vi "TestResult_Init.vi"(8 "error in (no error)":errorcluster, 9 "testStartedEventRef":refnum<user-event>, 10 "resultStatusChangedEventRef":refnum<user-event>, 11 "TestResult in":refnum<class "TestResult.lvclass">) -> (0 "error out":errorcluster, 3 "TestResult out":refnum<class "TestResult.lvclass">)   [LabVIEW 2013, in "TestResult.lvclass"]
uses:
  TestResult.lvclass
  resultStatusChanged--Cluster.ctl
  resultStatus--enum.ctl
  testStarted--Cluster.ctl
  private/testsRun.ctl
  private/shouldStop.ctl
  private/errors.ctl
  private/error.ctl
  private/failure.ctl
  TestResult.lvclass/TestResult.ctl
panel:
  # "JKI VI Tester for LabVIEW\nhttp://jkisoft.com/vi-tester\nCopyright (C) 2007-2009, JKI <info@jkisoft.com>\nALL RIGHTS RESERVED"
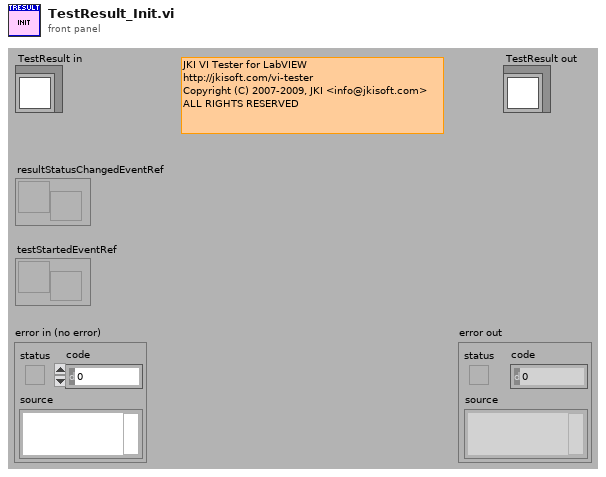
[diagram p1: front panel]
types:
  T1 = typedef "TestResult.lvclass/failure.ctl" = cluster{"test":refnum<class>, "error":errorcluster}
  T2 = typedef "TestResult.lvclass/errors.ctl" = T3[]
  T3 = typedef "TestResult.lvclass/error.ctl" = cluster{"test":refnum<class>, "error":errorcluster}
  T4 = typedef "TestResult.lvclass/shouldStop.ctl" = bool
  T5 = typedef "TestResult.lvclass/testsRun.ctl" = u32
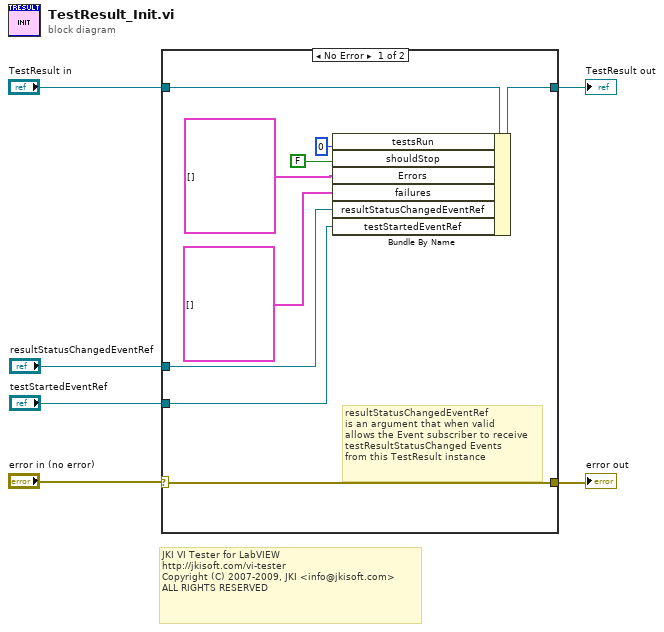
[diagram p0: block diagram]
diagram:
  # "JKI VI Tester for LabVIEW\nhttp://jkisoft.com/vi-tester\nCopyright (C) 2007-2009, JKI <info@jkisoft.com>\nALL RIGHTS RESERVED"
  n1 = case shown="No Error" "error in (no error)" {
    selector: "error in (no error)" -> [w13 w16]
    tunnel: "TestResult in" -> [w15 w17]
    tunnel: [w14 w17] -> w5
    tunnel: [w13 w16] -> w3
    tunnel: "resultStatusChangedEventRef" -> [w8 _]
    tunnel: "testStartedEventRef" -> [w7 _]
    frame No Error {
      # "resultStatusChangedEventRef\nis an argument that when valid\nallows the Event subscriber to receive\ntestResultStatusChanged Events\nfrom this TestResult instance"
      n2 = Bundle By Name(cluster=w15, "testsRun"=T5 0, "shouldStop"=T4 FALSE, "Errors"=T2 [], "failures"=T1[] [], "resultStatusChangedEventRef"=w8, "testStartedEventRef"=w7) -> (w14:refnum<class "TestResult.lvclass">)
    }
    frame Error {
    }
  }
  "TestResult out" <- w5
  "error out" <- w3
